vi "View.vi"() -> ()   [LabVIEW 2018]
doc: "Gestisce le interazioni dell'utente con l'interfaccia, genera gli stati corretti e li manda al controller."
uses:
  MessageCluster.ctl
panel:
  in  "Temperatura acqua doccia (°C)":u8(knob) scale=0.0..40.0
  out "Stato doccia":string
  out "stato doccia":bool
  in  "Doccia off/on":bool
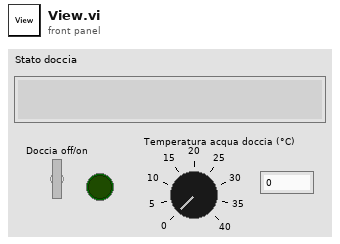
[diagram p1: front panel]
types:
  T1 = enum16{"On", "Off", "Preparation", "WaitTimer", "Ready"}
  T2 = typedef "MessageCluster.ctl" = cluster{"Message":string, "Temp":i32, "Stato":enum16{"On", "Off", "Preparation", "WaitTimer", "Ready"}}
  T3 = typedef "Messages.ctl" = string
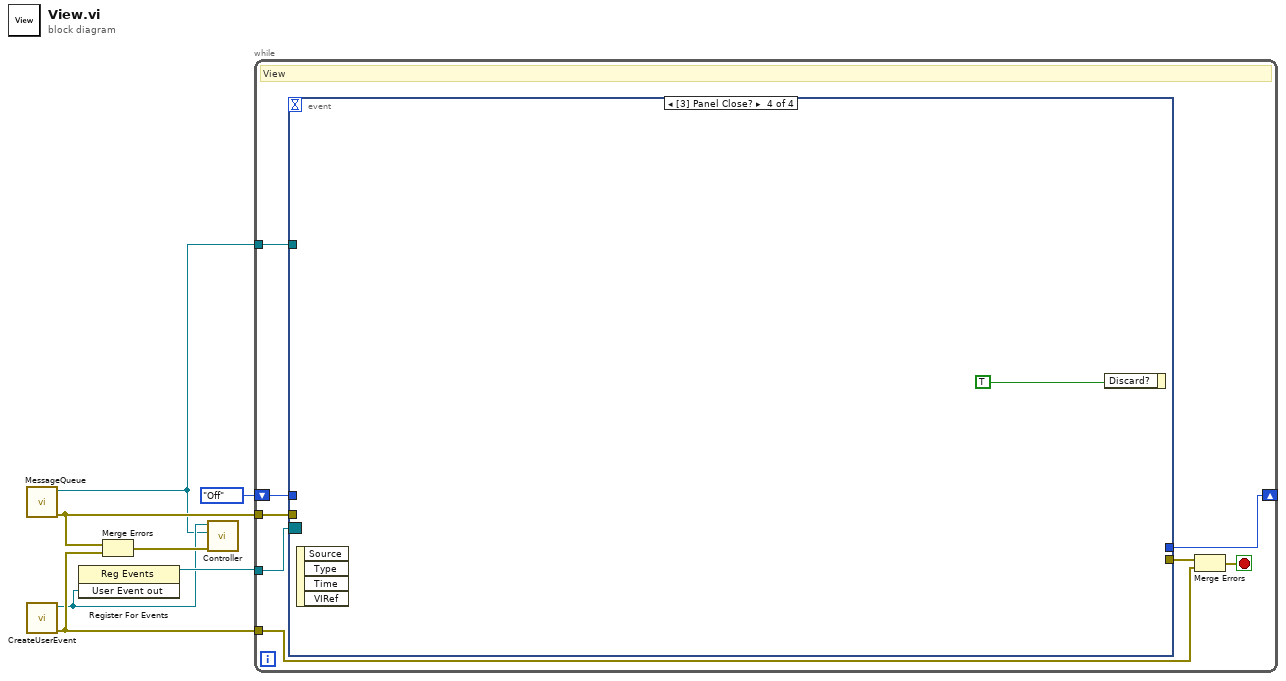
[diagram p0: block diagram]
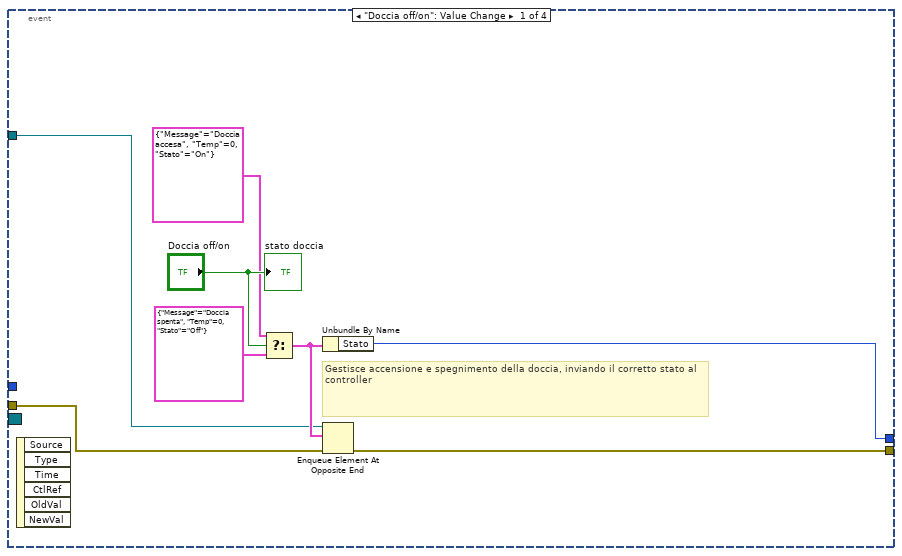
[diagram p2: hidden frame]
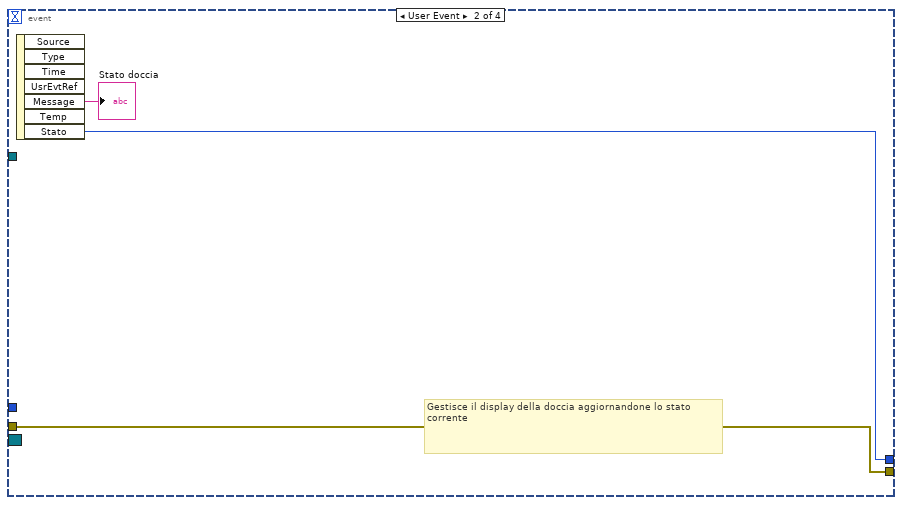
[diagram p3: hidden frame]
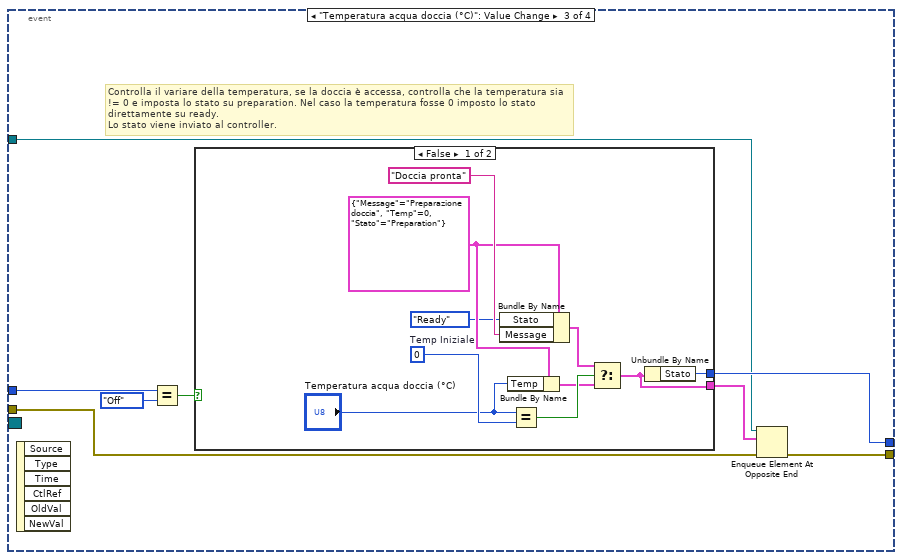
[diagram p4: hidden frame]
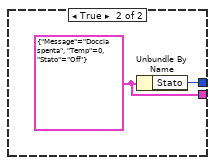
[diagram p5: hidden frame]
diagram:
  n1 = call "MessageQueue.vi"() -> ("error out"=w6:errorcluster, "Queue out"=w1:refnum<queue>)  [unwired: 10 in]
  n2 = call "CreateUserEvent.vi"() -> ("error out"=w4:errorcluster, "User Event out"=w2:refnum<user-event>)  [unwired: 10 in]
  n3 = register-events(w2) -> (reference out=w7:refnum<event-registration>)  [unwired: 2 in, 1 out]
  n4 = Merge Errors(w6, w4) -> (w5:errorcluster)
  n5 = call "Controller.vi"("User Event in"=w2, "State"=w1, "error in (state)"=w5) -> ()  [unwired: 8 in]
  n6 = while {
    shift-right: [w14] -> _
    shift-left: T1."Off" -> [w15]
    tunnel: w6 -> [w13]
    tunnel: w7 -> [w12]
    tunnel: w4 -> [w11]
    tunnel: w1 -> [w8]
    stop <- w9 stop-if-true
    # "View"
    n7 = event shown="[3] Panel Close?" {
      selector: w12 -> [_ _ _ _]
      dyn-events: _ -> [_ _ _ _]
      timeout: _ -> [_ _ _ _]
      tunnel: w15 -> [_ _ w33 _]
      tunnel: [w22 w25 w32 _] -> w14
      tunnel: w13 -> [w20 w26 w30 _]
      tunnel: [w19 w26 w29 _] -> w10
      tunnel: w8 -> [w18 _ w28 _]
      event "Doccia off/on": Value Change {
        # "Gestisce accensione e spegnimento della doccia, inviando il corretto stato al controller"
        n8 = event-data() -> ()  [unwired: 1 in, 6 out]
        n9 = Select(t=T2 {"Message"="Doccia accesa", "Temp"=0, "Stato"=enum."On"} ("Message Cluster"), s="Doccia off/on", f=T2 {"Message"="Doccia spenta", "Temp"=0, "Stato"=enum."Off"} ("Message Cluster")) -> (s? t:f=w21:T2)
        n10 = Unbundle By Name(w21) -> ("Stato"=w22:T1)
        n11 = Enqueue Element At Opposite End(queue=w18, element=w21, error in (no error)=w20) -> (error out=w19:errorcluster)  [unwired: 1 in, 2 out]
        "stato doccia" <- "Doccia off/on"
      }
      event User Event {
        # "Gestisce il display della doccia aggiornandone lo stato corrente"
        n12 = event-data() -> ("Message"=→"Stato doccia":T3, "Stato"=w25:T1)  [unwired: 1 in, 5 out]
      }
      event "Temperatura acqua doccia (°C)": Value Change {
        # "Controlla il variare della temperatura, se la doccia è accessa, controlla che la temperatura sia != 0 e imposta lo stato su preparation. Nel caso la temperatura fosse 0 imposto lo stato direttamente su ready.\nLo stato viene inviato al controller."
        n13 = event-data() -> ()  [unwired: 1 in, 6 out]
        n14 = Equal?(x=w33, y=enum16{"On", "Off", "Preparation", "Ready"}."Off") -> (x = y?=w34:bool)
        n15 = case shown="False" w34 {
          tunnel: [w37 w46] -> w32
          tunnel: [w38 w45] -> w27
          frame False {
            w36 = T2 {"Message"="Preparazione doccia", "Temp"=0, "Stato"=enum."Preparation"} ("Message Cluster")
            w44 = 0  # Temp Iniziale
            n16 = Bundle By Name(cluster=w36, "Stato"=T1."Ready", "Message"="Doccia pronta") -> (w39:T2)
            n17 = Bundle By Name(cluster=w36, "Temp"="Temperatura acqua doccia (°C)") -> (w41:T2)
            n18 = Equal?(x="Temperatura acqua doccia (°C)", y=w44) -> (x = y?=w43:bool)
            n19 = Select(t=w39, s=w43, f=w41) -> (s? t:f=w38:T2)
            n20 = Unbundle By Name(w38) -> ("Stato"=w37:T1)
          }
          frame True {
            w45 = T2 {"Message"="Doccia spenta", "Temp"=0, "Stato"=enum."Off"} ("Message Cluster")
            n21 = Unbundle By Name(w45) -> ("Stato"=w46:T1)
          }
        }
        n22 = Enqueue Element At Opposite End(queue=w28, element=w27, error in (no error)=w30) -> (error out=w29:errorcluster)  [unwired: 1 in, 2 out]
      }
      event Panel Close? {
        n23 = event-data() -> ()  [unwired: 1 in, 4 out]
        n24 = event-data("Discard?"=TRUE) -> ()  [unwired: 1 in, 1 out]
      }
    }
    n25 = Merge Errors(w10, w11) -> (w9:errorcluster)
  }
